vi "OnGetResourceHandlerEvent.vi"(4 "User Parameter":variant, 5 "Event Data":cluster{"sender":refnum<k24>, "e":refnum<k24>}, 6 "Control Ref":refnum<k24>, 7 "Event Common Data":T1) -> ()   [LabVIEW 2013]
uses:
  E:/Dropbox/ni/lvcef/github/lvcef/dotnet/LVCef/bin/Debug/LVCef.dll
  dotnet/LVCef/bin/Debug/LVCef.dll
  E:/Dropbox/ni/lvcef/github/lvcef/dotnet/LVCef/bin/Debug/Xilium.CefGlue.dll
  dotnet/LVCef/bin/Debug/Xilium.CefGlue.dll
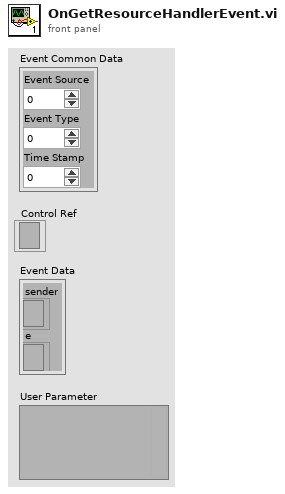
[diagram p1: front panel]
types:
  T1 = cluster{"Event Source":i32, "Event Type":u32, "Time Stamp":u32}
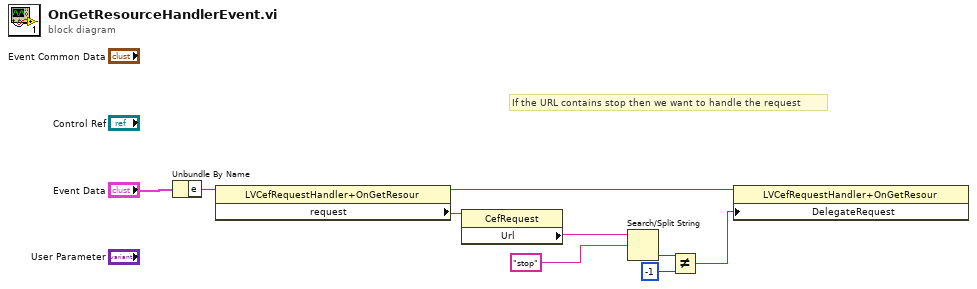
[diagram p0: block diagram]
diagram:
  # "If the URL contains stop then we want to handle the request"
  n1 = Unbundle By Name("Event Data") -> ("e"=w8:refnum<k24>)
  n2 = property class="LVCefRequestHandler+OnGetResour"(reference=w8) -> (reference out=w2:refnum<k24>, "request"=w7:refnum<k24>)  [unwired: 1 in, 1 out]
  n3 = property class="CefRequest"(reference=w7) -> ("Url"=w6:string)  [unwired: 1 in, 2 out]
  n4 = Search/Split String(string=w6, search string/char (-)="stop") -> (offset of match=w4:i32)  [unwired: 1 in, 2 out]
  n5 = Not Equal?(x=w4, y=-1) -> (x != y?=w1:bool)
  n6 = property class="LVCefRequestHandler+OnGetResour"(reference=w2, "DelegateRequest"=w1) -> ()  [unwired: 1 in, 2 out]
